vi "[Template]_Data To ASCII String.vi"(8 "error in":errorcluster, 11 "Data":i32[][](array[numeric])) -> (0 "error out":errorcluster, 3 "strings":string[](array[string]))   [LabVIEW 2016]
doc: "This VI takes data and converts it into an ASCII string. This VI must perform the opposite operation to the ASCIIStringToData function."
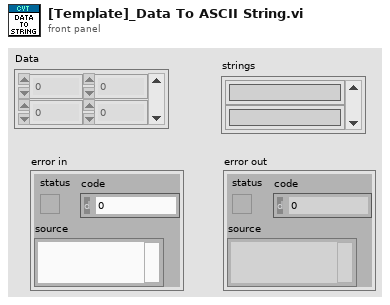
[diagram p1: front panel]
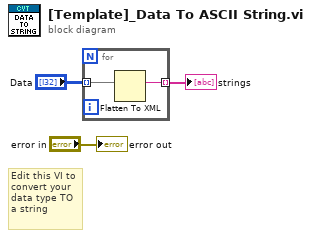
[diagram p0: block diagram]
diagram:
  # "Edit this VI to\nconvert your \ndata type TO\na string"
  n1 = for {
    tunnel: "Data" -> [w5] mode=indexing
    tunnel: [w4] -> w2 mode=indexing
    n2 = Flatten To XML(anything=w5) -> (xml string=w4:string)
  }
  "strings" <- w2
  "error out" <- "error in"
